vi "Get Position SubVi.vi"(0 "reference in":refnum<k24>, 1 "error in":errorcluster) -> (2 "reference out":refnum<k24>, 3 "error out":errorcluster, 4 "Current X Position":dbl[](array[numeric]), 5 "Current Y Position":dbl[](array[numeric]))   [LabVIEW 2017]
uses:
  Newport.XPS.CommandInterface
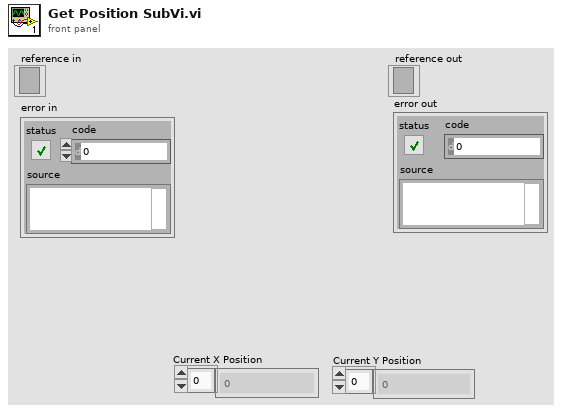
[diagram p1: front panel]
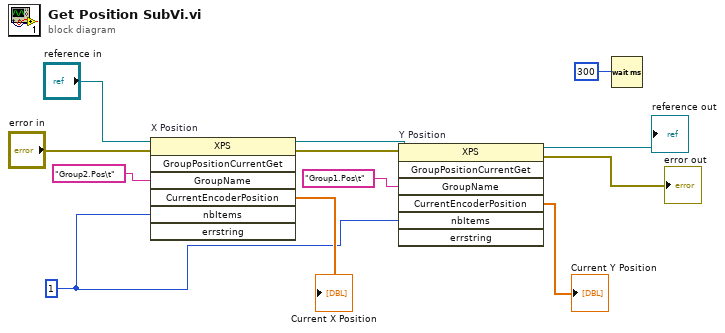
[diagram p0: block diagram]
diagram:
  w6 = 1
  n1 = invoke on="X Position" class="XPS" method="GroupPositionCurrentGet"(reference="reference in", error in="error in", "GroupName"="Group2.Pos\t", "nbItems"=w6) -> (reference out=w7:refnum<k24>, error out=w8:errorcluster, "CurrentEncoderPosition"=→"Current X Position":dbl[])  [unwired: 3 in, 4 out]
  n2 = invoke on="Y Position" class="XPS" method="GroupPositionCurrentGet"(reference=w7, error in=w8, "GroupName"="Group1.Pos\t", "nbItems"=w6) -> (reference out=→"reference out":refnum<k24>, error out=→"error out":errorcluster, "CurrentEncoderPosition"=→"Current Y Position":dbl[])  [unwired: 3 in, 4 out]
  n3 = Wait (ms)(milliseconds to wait=300) -> ()  [unwired: 1 out]
